vi "Read.vi"(8 "error in (no error)":errorcluster caption="entrée d'erreur (pas d'erreur)", 11 "Class UART Nodon.lvclass En entrée":refnum<class "Class UART Nodon.lvclass">) -> (0 "error out":errorcluster caption="sortie d'erreur", 3 "Class UART Nodon.lvclass En sortie":refnum<class "Class UART Nodon.lvclass">)   [LabVIEW 2020, in "Library Instrument & Equipement.lvlib" / "Library UART.lvlib" / "Class UART Nodon.lvclass"]
uses:
  Class UART Nodon.lvclass
  C:/Users/ngarcin/OneDrive - Altyor/Standard TB/Class/UART/UART (Default)/Class UART (Default).lvclass
  Class UART Nodon.lvclass/Class UART Nodon.ctl
  Commun VI/Library Commun.lvlib
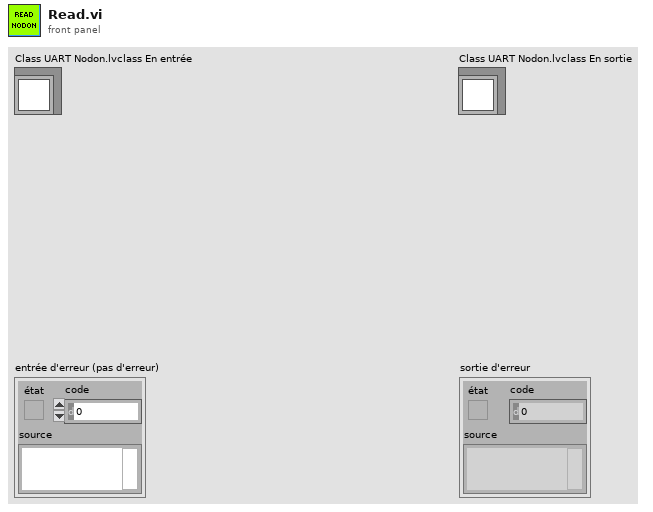
[diagram p1: front panel]
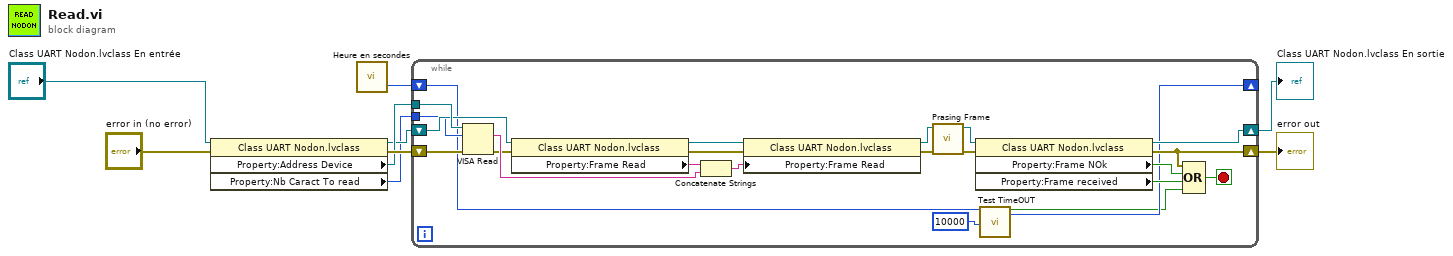
[diagram p0: block diagram]
diagram:
  n1 = property class="Class UART Nodon.lvclass"(reference="Class UART Nodon.lvclass En entrée", error in="error in (no error)") -> (reference out=w4:refnum<class "Class UART Nodon.lvclass">, error out=w6:errorcluster, "Property:Address Device"=w5:refnum<visa-resource-name>, "Property:Nb Caract To read"=w2:u32)
  n2 = call "Heure en secondes.vi"() -> ("Heure en milisecondes"=w1:u32)  [unwired: 2 in, 1 out]
  n3 = while {
    tunnel: w5 -> [w27]
    shift-right: [w15] -> w9
    shift-left: w6 -> [w28]
    shift-right: [w16] -> w8
    shift-left: w4 -> [w25]
    tunnel: w2 -> [w14]
    shift-right: [w11] -> _
    shift-left: w1 -> [w13]
    stop <- w26 stop-if-true
    n4 = VISA Read(VISA resource name=w27, byte count=w14, error in (no error)=w28) -> (read buffer=w21:string, error out=w17:errorcluster)  [unwired: 2 out]
    n5 = property class="Class UART Nodon.lvclass"(reference=w25, error in=w17) -> (reference out=w24:refnum<class "Class UART Nodon.lvclass">, error out=w23:errorcluster, "Property:Frame Read"=w22:string)
    n6 = Concatenate Strings(w22, w21) -> (w20:string)
    n7 = property class="Class UART Nodon.lvclass"(reference=w24, error in=w23, "Property:Frame Read"=w20) -> (reference out=w18:refnum<class "Class UART Nodon.lvclass">, error out=w19:errorcluster)
    n8 = call-dynamic "Prasing Frame.vi"("error in (no error)"=w19, "Class UART Nodon.lvclass En entrée"=w18) -> ("error out"=w31:errorcluster, "Class UART Nodon.lvclass En sortie"=w32:refnum<class "Class UART Nodon.lvclass">)  [unwired: 8 in]
    n9 = property class="Class UART Nodon.lvclass"(reference=w32, error in=w31) -> (reference out=w16:refnum<class "Class UART Nodon.lvclass">, error out=w15:errorcluster, "Property:Frame NOk"=w30:bool, "Property:Frame received"=w29:bool)
    n10 = call "Test TimeOUT.vi"("OLD Time"=w13, "TimeOut ms"=u32 10000) -> ("Timeout ?"=w10:bool, "NEW Time"=w11:u32)  [unwired: 13 in, 3 out]
    n11 = Compound Arithmetic op=OR ("Opérateur arithmétique")(w15, w30, w29, w10) -> (w26:bool)
  }
  "error out" <- w9
  "Class UART Nodon.lvclass En sortie" <- w8
